vi "Configure Resistance Voltage Source.vi"(7 "Voltage Source Value (0: Voltage Source Setting Value)":i32(ring) items=["Voltage Source Setting Value", "Measured Source Value"], 8 "error in (no error)":errorcluster, 9 "Voltage Source Control (0: Manual)":i32(ring) items=["Manual", "Auto"], 10 "Channel (1: Channel 1)":i32(ring)=1 items=["Channel 1"=1, "Channel 2"=2], 11 "VISA resource name":refnum<visa-resource-name>) -> (0 "error out":errorcluster, 3 "VISA resource name out":refnum<visa-resource-name>)   [LabVIEW 2012, in "Keysight B2980 Series.lvlib"]
doc: "Configures the voltage source control and value for resistance measurement.\n\n<b>Note(s):</b>\nThis VI is only applicable for model B2985A and B2987A."
uses:
  Keysight B2980 Series.lvlib
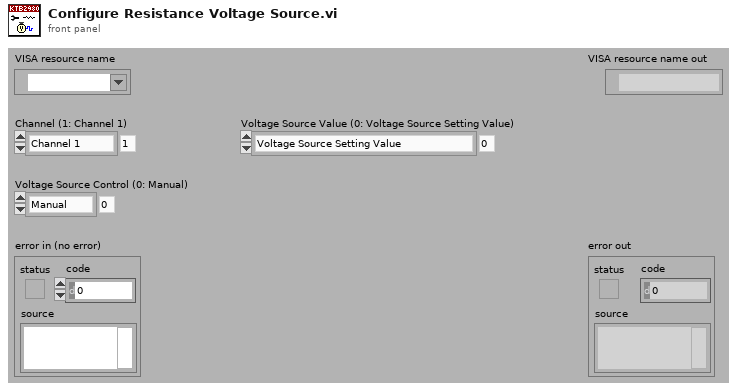
[diagram p1: front panel]
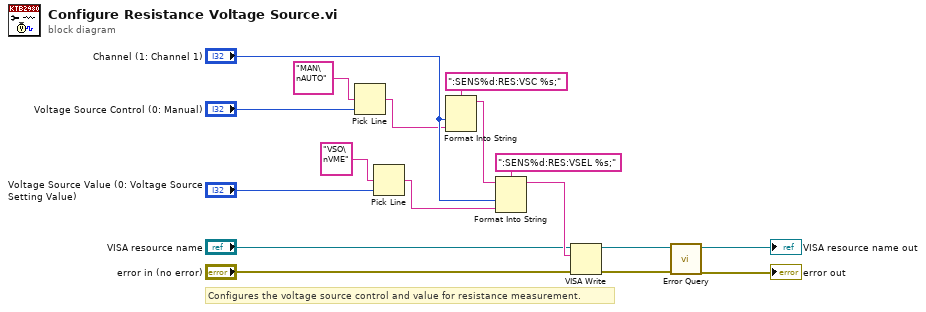
[diagram p0: block diagram]
diagram:
  # "Configures the voltage source control and value for resistance measurement."
  n1 = Pick Line(multi-line string="MAN\nAUTO", line index="Voltage Source Control (0: Manual)") -> (output string=w13:string)  [unwired: 1 out]
  n2 = Pick Line(multi-line string="VSO\nVME", line index="Voltage Source Value (0: Voltage Source Setting Value)") -> (output string=w8:string)  [unwired: 1 out]
  n3 = Format Into String(format string=":SENS%d:RES:VSC %s;", "Channel (1: Channel 1)", w13) -> (resulting string=w10:string)  [unwired: 2 in, 1 out]
  n4 = Format Into String(format string=":SENS%d:RES:VSEL %s;", initial string=w10, "Channel (1: Channel 1)", w8) -> (resulting string=w7:string)  [unwired: 1 in, 1 out]
  n5 = VISA Write(VISA resource name="VISA resource name", write buffer=w7, error in (no error)="error in (no error)") -> (VISA resource name out=w4:refnum<visa-resource-name>, error out=w3:errorcluster)  [unwired: 1 out]
  n6 = call "Error Query.vi"("error in (no error)"=w3, "VISA resource name"=w4) -> ("error out"=→"error out":errorcluster, "VISA resource name out"=→"VISA resource name out":refnum<visa-resource-name>)  [unwired: 8 out]
